vi "PulseTrain (G3)-Init PWM.vi"(0 "Pulse Rate (Hz)":dbl, 5 "Phase (cycles)":dbl, 7 "Fs (Hz)":dbl, 9 "Npts":i32, 11 "error in (no error)":errorcluster, 12 "Duty cycle":dbl) -> (4 "Initial State":T1, 15 "error out":errorcluster)   [LabVIEW 2015]
uses:
  Pulse Train-PWM State.ctl
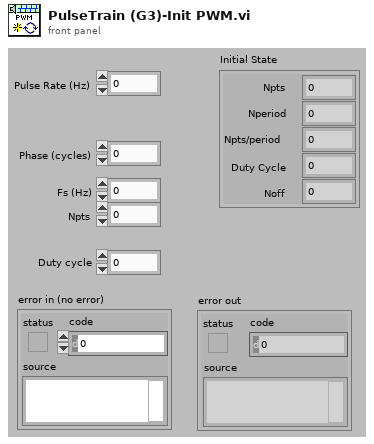
[diagram p1: front panel]
types:
  T1 = typedef "Pulse Train-PWM State.ctl" = cluster{"Npts":i32, "Nperiod":i32, "Npts/period":i32, "Duty Cycle":dbl, "Noff":i32}
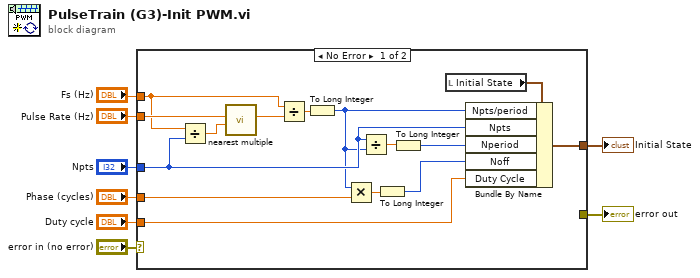
[diagram p0: block diagram]
diagram:
  n1 = case shown="No Error" "error in (no error)" {
    selector: "error in (no error)" -> [_ w24]
    tunnel: [_ w24] -> w7
    tunnel: "Fs (Hz)" -> [w18 _]
    tunnel: [w22 _] -> w5
    tunnel: "Pulse Rate (Hz)" -> [w21 _]
    tunnel: "Phase (cycles)" -> [w16 _]
    tunnel: "Npts" -> [w13 _]
    tunnel: "Duty cycle" -> [w9 _]
    frame No Error {
      n2 = Divide(x=w18, y=w13) -> (x/y=w20:dbl)
      n3 = call "nearest multiple.vi"("y"=w20, "x"=w21) -> ("round(x/y)*y"=w19:dbl)  [unwired: 7 in, 2 out]
      n4 = Divide(x=w18, y=w19) -> (x/y=w17:dbl)
      n5 = To Long Integer(number=w17) -> (32bit integer=w12:i32)
      n6 = Multiply(x=w12, y=w16) -> (x*y=w15:dbl)
      n7 = Divide(x=w13, y=w12) -> (x/y=w11:dbl)
      n8 = To Long Integer(number=w15) -> (32bit integer=w14:i32)
      n9 = To Long Integer(number=w11) -> (32bit integer=w10:i32)
      n10 = local read "Initial State"() -> (w23:T1)
      n11 = Bundle By Name(cluster=w23, "Npts/period"=w12, "Npts"=w13, "Nperiod"=w10, "Noff"=w14, "Duty Cycle"=w9) -> (w22:T1)
    }
    frame Error {
    }
  }
  "error out" <- w7
  "Initial State" <- w5
